vi "helpme.vi"(11 "Numeric":dbl) -> ()   [LabVIEW 2014]
uses:
  <vilib>/Rock Robotics/WPI/Solenoid/WPI_SolenoidValue.ctl
  <vilib>/Rock Robotics/WPI/Solenoid/WPI_SolenoidSetEnum.vi
  Robot Global Data.vi
  <vilib>/Rock Robotics/WPI/RobotDrive/WPI_RobotDriveGetSetRefNum.vi
  <vilib>/Rock Robotics/WPI/RobotDrive/WPI_RobotDriveMecanumDrive_Cartesian.vi
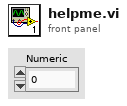
[diagram p1: front panel]
types:
  T1 = typedef "WPI_SolenoidValue.ctl" = enum16{"Off", "On", "Forward", "Reverse"}
  T2 = typedef "WPI_GyroDevRef.ctl" = cluster{"DevStatus":errorcluster, "Analog Module":T3, "Analog Channel":T4, "Offset":dbl, "Gain (VoltsPerDegree/Second)":dbl}
  T3 = typedef "FPGA_TypedefAnalogModule.ctl" = enum16{"Controller 1"}
  T4 = typedef "FPGA_AIChannel.ctl" = enum8{"AI 0", "AI 1", "AI 2", "AI 3", "AI MXP 0", "AI MXP 1", "AI MXP 2", "AI MXP 3", "Invalid"}
  T5 = typedef "WPI_SolenoidDevRef.ctl" = cluster{"DevStatus":errorcluster, "Pneumatics Control Module":u8, "Forward Solenoid Channel":T6, "Reverse Solenoid Channel":T6}
  T6 = typedef "WPI_SolenoidChannel.ctl" = enum8{"Solenoid 0", "Solenoid 1", "Solenoid 2", "Solenoid 3", "Solenoid 4", "Solenoid 5", "Solenoid 6", "Solenoid 7", "Invalid"}
  T7 = typedef "WPI_MotorControlDeviceRef.ctl" = cluster{"DeviceStatus":errorcluster, "Type":T8, "PWM":cluster{"Controller":T9, "PWM Channel":T10, "DeadBand":T11}, "CAN":cluster{"Device Number":u8, "Control Mode":T12, "Semaphore":T13, "Max Vout":dbl, "TalonSRX Control Mode":T14}, "Invert":bool, "TransformRef":T15, "InvTransformRef":T15}
  T8 = typedef "WPI_MotorControlType.ctl" = enum16{"PWM", "CAN", "CANTalonSRX"}
  T9 = typedef "FPGA_TypedefDigitalModule.ctl" = enum16{"Controller 1"}
  T10 = typedef "FPGA_DIOPWMChannel.ctl" = enum8{"PWM 0", "PWM 1", "PWM 2", "PWM 3", "PWM 4", "PWM 5", "PWM 6", "PWM 7", "PWM 8", "PWM 9", "PWM MXP 0", "PWM MXP 1", "PWM MXP 2", "PWM MXP 3", "PWM MXP 4", "PWM MXP 5", "PWM MXP 6", "PWM MXP 7", "PWM MXP 8", "PWM MXP 9", "Invalid"}
  T11 = typedef "WPI_PWMDeadband.ctl" = cluster{"Name":string, "maxPositivePwm":i32, "minPositivePwm":i32, "centerPwm":i32, "maxNegativePwm":i32, "minNegativePwm":i32, "angularRange":u16}
  T12 = typedef "WPI_CANJaguar_ControlMode.ctl" = enum8{"Percent VBus", "Current", "Speed", "Position", "Voltage"}
  T13 = typedef "Semaphore RefNum" = refnum<k1>
  T14 = typedef "WPI_CANTalonSRX_APIControlMode.ctl" = enum8{"Percent VBus", "Speed", "Position", "Slave", "Unchanged / Invalid"}
  T15 = typedef "WPI_PWMTransform_ConPane.ctl" = refnum<vi>
  T16 = typedef "WPI_RobotDriveDevRef.ctl" = cluster{"DevStatus":errorcluster, "Motors[]":T7[], "Square Inputs":bool, "Max Output":dbl}
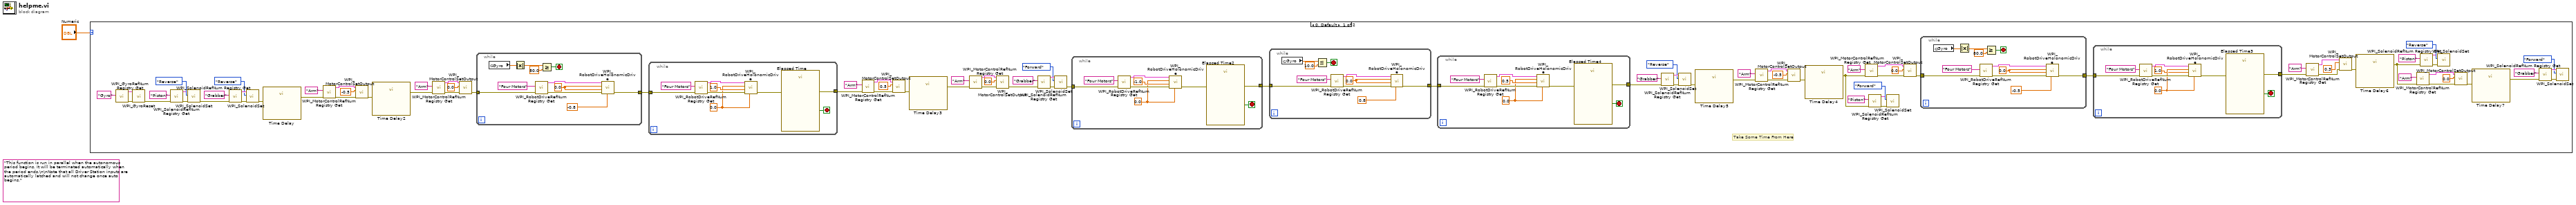
[diagram p0: block diagram]
diagram:
  (unwired) "This function is run in parallel when the autonomous period begins. It will be terminated automatically when the period ends.\n\nNote that all Driver Station inputs are automatically latched and will not change once auto begins."
  n1 = case shown="0, Default" "Numeric" {
    frame 0, Default {
      # "Take Some Time From Here"
      n2 = call <vilib>:"WPI_GyroRefNum Registry Get.vi"("refnum name"="Gyro") -> ("error out"=w67:errorcluster, "GyroDevRef"=w68:T2)  [unwired: 9 in]
      n3 = call <vilib>:"WPI_GyroReset.vi"("error in (no error)"=w67, "GyroDevRef"=w68) -> ("error out"=w65:errorcluster)  [unwired: 8 in, 1 out]
      n4 = call <vilib>:"WPI_SolenoidRefNum Registry Get.vi"("error in (no error)"=w65, "refnum name"="Piston") -> ("error out"=w85:errorcluster, "SolenoidDevRef"=w86:T5)  [unwired: 8 in]
      n5 = call-poly <vilib>:"WPI_SolenoidSet.vi"("error in (no error)"=w85, "Value"=WPI_SolenoidValue."Reverse", "SolenoidDevRef"=w86) -> ("error out"=w83:errorcluster)  [unwired: 7 in, 1 out]
      n6 = call <vilib>:"WPI_SolenoidRefNum Registry Get.vi"("error in (no error)"=w83, "refnum name"="Grabber") -> ("error out"=w90:errorcluster, "SolenoidDevRef"=w89:T5)  [unwired: 8 in]
      n7 = call-poly <vilib>:"WPI_SolenoidSet.vi"("error in (no error)"=w90, "Value"=WPI_SolenoidValue."Reverse", "SolenoidDevRef"=w89) -> ("error out"=w82:errorcluster)  [unwired: 7 in, 1 out]
      n8 = call "Time Delay"("error in (no error)"=w82) -> ("error out"=w78:errorcluster)  [unwired: 10 in]
      n9 = call <vilib>:"WPI_MotorControlRefNum Registry Get.vi"("error in (no error)"=w78, "refnum name"="Arm") -> ("error out"=w81:errorcluster, "MotorControlDevRef"=w80:T7)  [unwired: 8 in]
      n10 = call <vilib>:"WPI_MotorControlSetOutput.vi"("error in (no error)"=w81, "Output"=-0.5, "MotorControlDevRef"=w80) -> ("error out"=w77:errorcluster)  [unwired: 6 in, 2 out]
      n11 = call "Time Delay2"("error in (no error)"=w77) -> ("error out"=w70:errorcluster)  [unwired: 10 in]
      n12 = call <vilib>:"WPI_MotorControlRefNum Registry Get.vi"("error in (no error)"=w70, "refnum name"="Arm") -> ("error out"=w71:errorcluster, "MotorControlDevRef"=w72:T7)  [unwired: 8 in]
      n13 = call <vilib>:"WPI_MotorControlSetOutput.vi"("error in (no error)"=w71, "Output"=0.0, "MotorControlDevRef"=w72) -> ("error out"=w69:errorcluster)  [unwired: 6 in, 2 out]
      n14 = while {
        tunnel: w69 -> [w158]
        tunnel: [w150] -> w75
        stop <- w154 stop-if-true
        w149 = 0.0 ("X")
        n15 = global read "Robot Global Data.vi" "Gyro"() -> (w151:dbl)
        n16 = Absolute Value(x=w151) -> (abs(x)=w152:dbl)
        n17 = call <vilib>:"WPI_RobotDriveRefNum Registry Get.vi"("error in (no error)"=w158, "refnum name"="Four Motors") -> ("error out"=w157:errorcluster, "RobotDriveDevRef"=w156:T16)  [unwired: 8 in]
        n18 = Greater Or Equal?(x=w152, y=80.0) -> (x >= y?=w154:bool)
        n19 = call-poly <vilib>:"WPI_RobotDriveHolonomicDrive.vi"("Rotation"=-0.8, "error in (no error)"=w157, "Y"=w149, "X"=w149, "RobotDriveDevRef"=w156) -> ("error out"=w150:errorcluster)  [unwired: 4 in, 2 out]
      }
      n20 = while {
        tunnel: w75 -> [w147]
        tunnel: [w140] -> w50
        stop <- w144 stop-if-true
        w141 = 0.0 ("Y")
        n21 = call <vilib>:"WPI_RobotDriveRefNum Registry Get.vi"("error in (no error)"=w147, "refnum name"="Four Motors") -> ("error out"=w146:errorcluster, "RobotDriveDevRef"=w145:T16)  [unwired: 8 in]
        n22 = call-poly <vilib>:"WPI_RobotDriveHolonomicDrive.vi"("Rotation"=w141, "error in (no error)"=w146, "Y"=1.0 ("Rotation"), "X"=w141, "RobotDriveDevRef"=w145) -> ("error out"=w143:errorcluster)  [unwired: 4 in, 2 out]
        n23 = call "Elapsed Time"("error in (no error)"=w143) -> ("Time has Elapsed"=w144:bool, "error out"=w140:errorcluster)  [unwired: 11 in, 6 out]
      }
      n24 = call <vilib>:"WPI_MotorControlRefNum Registry Get.vi"("error in (no error)"=w50, "refnum name"="Arm") -> ("error out"=w60:errorcluster, "MotorControlDevRef"=w59:T7)  [unwired: 8 in]
      n25 = call <vilib>:"WPI_MotorControlSetOutput.vi"("error in (no error)"=w60, "Output"=0.5, "MotorControlDevRef"=w59) -> ("error out"=w57:errorcluster)  [unwired: 6 in, 2 out]
      n26 = call "Time Delay3"("error in (no error)"=w57) -> ("error out"=w51:errorcluster)  [unwired: 10 in]
      n27 = call <vilib>:"WPI_MotorControlRefNum Registry Get.vi"("error in (no error)"=w51, "refnum name"="Arm") -> ("error out"=w52:errorcluster, "MotorControlDevRef"=w53:T7)  [unwired: 8 in]
      n28 = call <vilib>:"WPI_MotorControlSetOutput.vi"("error in (no error)"=w52, "Output"=0.0, "MotorControlDevRef"=w53) -> ("error out"=w49:errorcluster)  [unwired: 6 in, 2 out]
      n29 = call <vilib>:"WPI_SolenoidRefNum Registry Get.vi"("error in (no error)"=w49, "refnum name"="Grabber") -> ("error out"=w63:errorcluster, "SolenoidDevRef"=w62:T5)  [unwired: 8 in]
      n30 = call-poly <vilib>:"WPI_SolenoidSet.vi"("error in (no error)"=w63, "Value"=WPI_SolenoidValue."Forward", "SolenoidDevRef"=w62) -> ("error out"=w48:errorcluster)  [unwired: 7 in, 1 out]
      n31 = while {
        tunnel: [w134] -> w47
        tunnel: w48 -> [w131]
        stop <- w136 stop-if-true
        w132 = 0.0 ("Y")
        n32 = call <vilib>:"WPI_RobotDriveRefNum Registry Get.vi"("error in (no error)"=w131, "refnum name"="Four Motors") -> ("error out"=w138:errorcluster, "RobotDriveDevRef"=w137:T16)  [unwired: 8 in]
        n33 = call-poly <vilib>:"WPI_RobotDriveHolonomicDrive.vi"("Rotation"=w132, "error in (no error)"=w138, "Y"=-1.0 ("Rotation"), "X"=w132, "RobotDriveDevRef"=w137) -> ("error out"=w135:errorcluster)  [unwired: 4 in, 2 out]
        n34 = call "Elapsed Time2"("error in (no error)"=w135) -> ("Time has Elapsed"=w136:bool, "error out"=w134:errorcluster)  [unwired: 11 in, 6 out]
      }
      n35 = while {
        tunnel: w47 -> [w129]
        tunnel: [w125] -> w46
        stop <- w122 stop-if-true
        w124 = 0.0 ("Y")
        n36 = global read "Robot Global Data.vi" "Gyro"() -> (w121:dbl)
        n37 = Less Or Equal?(x=w121, y=10.0) -> (x <= y?=w122:bool)
        n38 = call <vilib>:"WPI_RobotDriveRefNum Registry Get.vi"("error in (no error)"=w129, "refnum name"="Four Motors") -> ("error out"=w128:errorcluster, "RobotDriveDevRef"=w127:T16)  [unwired: 8 in]
        n39 = call-poly <vilib>:"WPI_RobotDriveHolonomicDrive.vi"("Rotation"=0.8, "error in (no error)"=w128, "Y"=w124, "X"=w124, "RobotDriveDevRef"=w127) -> ("error out"=w125:errorcluster)  [unwired: 4 in, 2 out]
      }
      n40 = while {
        tunnel: [w95] -> w21
        tunnel: w46 -> [w92]
        stop <- w97 stop-if-true
        w93 = 0.0 ("Y")
        n41 = call <vilib>:"WPI_RobotDriveRefNum Registry Get.vi"("error in (no error)"=w92, "refnum name"="Four Motors") -> ("error out"=w99:errorcluster, "RobotDriveDevRef"=w98:T16)  [unwired: 8 in]
        n42 = call-poly <vilib>:"WPI_RobotDriveHolonomicDrive.vi"("Rotation"=w93, "error in (no error)"=w99, "Y"=0.5 ("Rotation"), "X"=w93, "RobotDriveDevRef"=w98) -> ("error out"=w96:errorcluster)  [unwired: 4 in, 2 out]
        n43 = call "Elapsed Time4"("error in (no error)"=w96) -> ("Time has Elapsed"=w97:bool, "error out"=w95:errorcluster)  [unwired: 11 in, 6 out]
      }
      n44 = call <vilib>:"WPI_SolenoidRefNum Registry Get.vi"("error in (no error)"=w21, "refnum name"="Grabber") -> ("error out"=w44:errorcluster, "SolenoidDevRef"=w43:T5)  [unwired: 8 in]
      n45 = call-poly <vilib>:"WPI_SolenoidSet.vi"("error in (no error)"=w44, "Value"=WPI_SolenoidValue."Reverse", "SolenoidDevRef"=w43) -> ("error out"=w27:errorcluster)  [unwired: 7 in, 1 out]
      n46 = call "Time Delay5"("error in (no error)"=w27) -> ("error out"=w20:errorcluster)  [unwired: 10 in]
      n47 = call <vilib>:"WPI_MotorControlRefNum Registry Get.vi"("error in (no error)"=w20, "refnum name"="Arm") -> ("error out"=w41:errorcluster, "MotorControlDevRef"=w40:T7)  [unwired: 8 in]
      n48 = call <vilib>:"WPI_MotorControlSetOutput.vi"("error in (no error)"=w41, "Output"=-0.5, "MotorControlDevRef"=w40) -> ("error out"=w38:errorcluster)  [unwired: 6 in, 2 out]
      n49 = call "Time Delay4"("error in (no error)"=w38) -> ("error out"=w2:errorcluster)  [unwired: 10 in]
      n50 = call <vilib>:"WPI_MotorControlRefNum Registry Get.vi"("error in (no error)"=w2, "refnum name"="Arm") -> ("error out"=w33:errorcluster, "MotorControlDevRef"=w34:T7)  [unwired: 8 in]
      n51 = call <vilib>:"WPI_SolenoidRefNum Registry Get.vi"("error in (no error)"=w2, "refnum name"="Piston") -> ("error out"=w23:errorcluster, "SolenoidDevRef"=w24:T5)  [unwired: 8 in]
      n52 = call-poly <vilib>:"WPI_SolenoidSet.vi"("error in (no error)"=w23, "Value"=WPI_SolenoidValue."Forward", "SolenoidDevRef"=w24) -> ()  [unwired: 7 in, 2 out]
      n53 = call <vilib>:"WPI_MotorControlSetOutput.vi"("error in (no error)"=w33, "Output"=0.0, "MotorControlDevRef"=w34) -> ("error out"=w28:errorcluster)  [unwired: 6 in, 2 out]
      n54 = while {
        tunnel: [w112] -> w26
        tunnel: w28 -> [w110]
        stop <- w116 stop-if-true
        w111 = 0.0 ("Y")
        n55 = global read "Robot Global Data.vi" "Gyro"() -> (w113:dbl)
        n56 = Absolute Value(x=w113) -> (abs(x)=w114:dbl)
        n57 = call <vilib>:"WPI_RobotDriveRefNum Registry Get.vi"("error in (no error)"=w110, "refnum name"="Four Motors") -> ("error out"=w119:errorcluster, "RobotDriveDevRef"=w118:T16)  [unwired: 8 in]
        n58 = Greater Or Equal?(x=w114, y=80.0) -> (x >= y?=w116:bool)
        n59 = call-poly <vilib>:"WPI_RobotDriveHolonomicDrive.vi"("Rotation"=-0.5, "error in (no error)"=w119, "Y"=w111, "X"=w111, "RobotDriveDevRef"=w118) -> ("error out"=w112:errorcluster)  [unwired: 4 in, 2 out]
      }
      n60 = while {
        tunnel: [w104] -> w10
        tunnel: w26 -> [w101]
        stop <- w106 stop-if-true
        w103 = 0.0 ("Y")
        n61 = call <vilib>:"WPI_RobotDriveRefNum Registry Get.vi"("error in (no error)"=w101, "refnum name"="Four Motors") -> ("error out"=w108:errorcluster, "RobotDriveDevRef"=w107:T16)  [unwired: 8 in]
        n62 = call-poly <vilib>:"WPI_RobotDriveHolonomicDrive.vi"("Rotation"=w103, "error in (no error)"=w108, "Y"=1.0 ("Rotation"), "X"=w103, "RobotDriveDevRef"=w107) -> ("error out"=w105:errorcluster)  [unwired: 4 in, 2 out]
        n63 = call "Elapsed Time3"("error in (no error)"=w105) -> ("Time has Elapsed"=w106:bool, "error out"=w104:errorcluster)  [unwired: 11 in, 6 out]
      }
      n64 = call <vilib>:"WPI_MotorControlRefNum Registry Get.vi"("error in (no error)"=w10, "refnum name"="Arm") -> ("error out"=w12:errorcluster, "MotorControlDevRef"=w13:T7)  [unwired: 8 in]
      n65 = call <vilib>:"WPI_MotorControlSetOutput.vi"("error in (no error)"=w12, "Output"=0.3, "MotorControlDevRef"=w13) -> ("error out"=w11:errorcluster)  [unwired: 6 in, 2 out]
      n66 = call "Time Delay6"("error in (no error)"=w11) -> ("error out"=w3:errorcluster)  [unwired: 10 in]
      n67 = call <vilib>:"WPI_MotorControlRefNum Registry Get.vi"("error in (no error)"=w3, "refnum name"="Arm") -> ("error out"=w8:errorcluster, "MotorControlDevRef"=w7:T7)  [unwired: 8 in]
      n68 = call <vilib>:"WPI_SolenoidRefNum Registry Get.vi"("error in (no error)"=w3, "refnum name"="Piston") -> ("error out"=w17:errorcluster, "SolenoidDevRef"=w18:T5)  [unwired: 8 in]
      n69 = call-poly <vilib>:"WPI_SolenoidSet.vi"("error in (no error)"=w17, "Value"=WPI_SolenoidValue."Reverse", "SolenoidDevRef"=w18) -> ()  [unwired: 7 in, 2 out]
      n70 = call <vilib>:"WPI_MotorControlSetOutput.vi"("error in (no error)"=w8, "Output"=0.0, "MotorControlDevRef"=w7) -> ("error out"=w4:errorcluster)  [unwired: 6 in, 2 out]
      n71 = call "Time Delay7"("error in (no error)"=w4) -> ("error out"=w9:errorcluster)  [unwired: 10 in]
      n72 = call <vilib>:"WPI_SolenoidRefNum Registry Get.vi"("error in (no error)"=w9, "refnum name"="Grabber") -> ("error out"=w31:errorcluster, "SolenoidDevRef"=w30:T5)  [unwired: 8 in]
      n73 = call-poly <vilib>:"WPI_SolenoidSet.vi"("error in (no error)"=w31, "Value"=WPI_SolenoidValue."Forward", "SolenoidDevRef"=w30) -> ()  [unwired: 7 in, 2 out]
    }
    frame 1 {
    }
  }
